vi "get channels.vi"(11 "user tag bus module configuration In":refnum<class "fixed channel tag bus module configuration.lvclass">) -> (2 "channels":refnum<class "TBM channel.lvclass">[](array[class]), 3 "user tag bus module configuration Out":refnum<class "fixed channel tag bus module configuration.lvclass">)   [LabVIEW 2013, in "fixed channel tag bus module configuration.lvclass"]
uses:
  fixed channel tag bus module configuration.lvclass
  <vilib>/NI/Tag Bus Module Framework/channel/TBM channel.lvclass
  fixed channel tag bus module configuration.lvclass/fixed channel tag bus module configuration.ctl
  <vilib>/NI/Tag Bus/tag/tag descriptor.lvclass/tag descriptor.ctl
  <vilib>/NI/Tag Bus/tag/read data type.vi
  <vilib>/NI/Tag Bus/tag/read tag name.vi
  <vilib>/NI/Tag Bus/tag/tag descriptor.lvclass
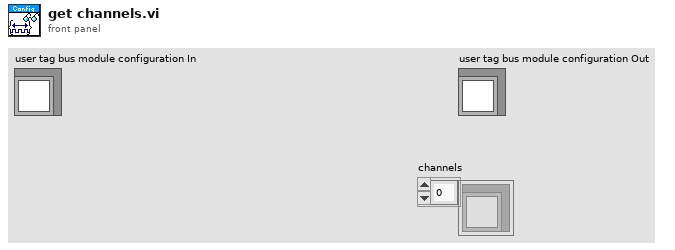
[diagram p1: front panel]
types:
  T1 = typedef "tag bus.lvlib/tag descriptor.lvclass/Data Type.ctl" = enum16{"Double", "Single", "I64", "I32", "I16", "I8", "U64", "U32", "U16", "U8", "Boolean", "String", "Array of Double", "Array of Single", "Array of I64", "Array of I32", "Array of I16", "Array of I8", "Array of U64", "Array of U32", "Array of U16", "Array of U8", "Array of Boolean", "Array of String"}
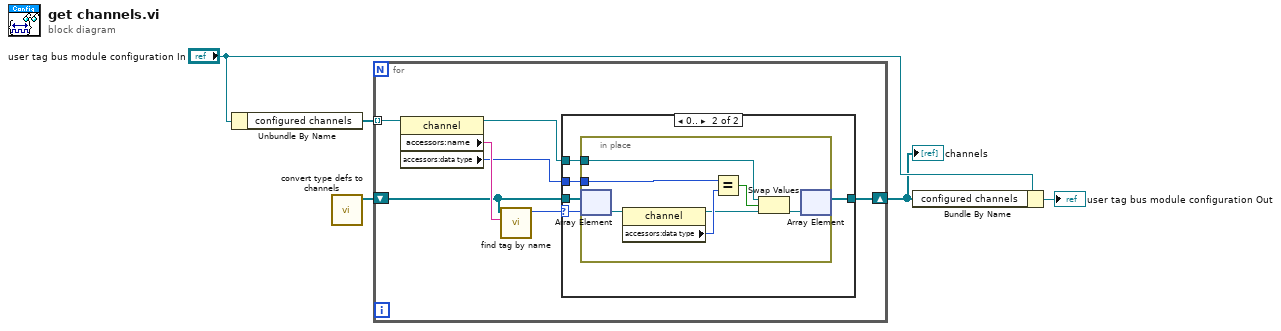
[diagram p0: block diagram]
diagram:
  n1 = Unbundle By Name("user tag bus module configuration In") -> ("configured channels"=w1:refnum<class "TBM channel.lvclass">[])
  n2 = call "convert type defs to channels.vi"() -> ("Array out"=w3:refnum<class "TBM channel.lvclass">[])  [unwired: 10 in, 1 out]
  n3 = for {
    shift-right: [w8] -> w2
    shift-left: w3 -> [w9]
    tunnel: w1 -> [w12] mode=indexing
    n4 = property class="channel"(reference=w12) -> (reference out=w6:refnum<class "TBM channel.lvclass">, "accessors:name"=w11:string, "accessors:data type"=w7:T1)  [unwired: 1 in, 1 out]
    n5 = call <vilib>:"find tag by name.vi"("name"=w11, "tags in"=w9) -> ("index"=w10:i32)  [unwired: 9 in]
    n6 = case shown="0.." w10 {
      selector: w10 -> [_ w17]
      tunnel: w9 -> [w13 w18]
      tunnel: [w13 w16] -> w8
      tunnel: w7 -> [_ w15]
      tunnel: w6 -> [_ w14]
      frame ..-1 {
      }
      frame 0.. {
        n7 = in-place {
          in-place-border: w15 -> [w23]
          in-place-border: w14 -> [w20]
          n8 = in-place-array #1(w18, w17) -> (w25:refnum<class "TBM channel.lvclass">)
          n9 = property class="channel"(reference=w25) -> (reference out=w22:refnum<class "TBM channel.lvclass">, "accessors:data type"=w24:T1)  [unwired: 1 in, 1 out]
          n10 = Equal?(x=w23, y=w24) -> (x = y?=w19:bool)
          n11 = Swap Values(12:w20, 13:w19, 14:w22) -> (3:w21:refnum<class "TBM channel.lvclass">)  [unwired: 1 out]
          n12 = in-place-array #1(w21) -> (w16:refnum<class "TBM channel.lvclass">[])  [unwired: 1 out]
        }
      }
    }
  }
  "channels" <- w2
  n13 = Bundle By Name(cluster="user tag bus module configuration In", "configured channels"=w2) -> (→"user tag bus module configuration Out":refnum<class "fixed channel tag bus module configuration.lvclass">)
